vi "Msg Handler.vi"(10 "Msg":refnum<class "Msg.lvclass">, 11 "TEMPLATE Actor in":refnum<class "TEMPLATE Actor.lvclass">) -> (0 "Error out":errorcluster, 3 "TEMPLATE Actor out":refnum<class "TEMPLATE Actor.lvclass">)   [LabVIEW 2025, in "_Template.lvlib" / "Templates.lvlib" / "TEMPLATE Actor.lvlib" / "TEMPLATE Actor.lvclass"]
uses:
  TEMPLATE Actor.lvclass
  jettl/jettl/Msg/Msg.lvclass
  jettl/jettl/Actor/Actor/Actor.lvclass
  TEMPLATE Actor.lvclass/TEMPLATE Actor.ctl
  jettl/jettl/Actor/Actor.lvlib
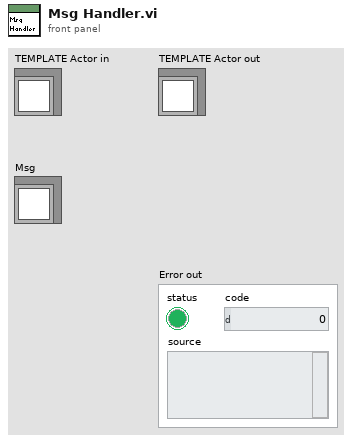
[diagram p1: front panel]
types:
  T1 = typedef "jettl.lvlib/Actor.lvlib/Msg Set.ctl" = set{refnum<class "Msg.lvclass">}
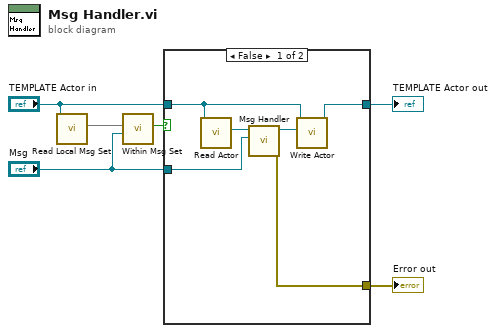
[diagram p0: block diagram]
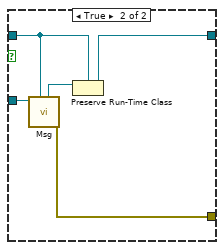
[diagram p2: hidden frame]
diagram:
  n1 = call-dynamic "Read Local Msg Set.vi"("TEMPLATE Actor in"="TEMPLATE Actor in") -> ("Local Msg Set"=w1:T1)  [unwired: 10 in]
  n2 = call "Within Msg Set.vi"("Msg"="Msg", "Msg Set"=w1) -> ("Within Msg Set"=w6:bool)  [unwired: 9 in]
  n3 = case shown="False" w6 {
    tunnel: "TEMPLATE Actor in" -> [w10 w15]
    tunnel: [w9 w14] -> w5
    tunnel: "Msg" -> [w12 w17]
    tunnel: [w11 w13] -> w3
    frame False {
      n4 = call-dynamic "Read Actor.vi"("TEMPLATE Actor in"=w10) -> ("Actor"=w8:refnum<class "Actor.lvclass">)  [unwired: 10 in]
      n5 = call-dynamic "Msg Handler.vi"("Msg"=w12, "Actor in"=w8) -> ("Error out"=w11:errorcluster, "Actor out"=w7:refnum<class "Actor.lvclass">)  [unwired: 8 in]
      n6 = call-dynamic "Write Actor.vi"("Actor"=w7, "TEMPLATE Actor in"=w10) -> ("TEMPLATE Actor out"=w9:refnum<class "TEMPLATE Actor.lvclass">)  [unwired: 9 in]
    }
    frame True {
      n7 = call-dynamic "Msg.vi"("Actor in"=w15, "Msg in"=w17) -> ("Error out"=w13:errorcluster, "Actor out"=w16:refnum<class "Actor.lvclass">)  [unwired: 8 in]
      n8 = Preserve Run-Time Class(object in=w16, 2:w15) -> (object out=w14:refnum<class "TEMPLATE Actor.lvclass">)  [unwired: 1 in, 1 out]
    }
  }
  "TEMPLATE Actor out" <- w5
  "Error out" <- w3
